vi "Sensors.vi"() -> ()   [LabVIEW 2017]
panel:
  in  "desired temp":dbl
  out "inside":dbl
  out "Gas":dbl
  out "Smoke":dbl
  out "Temp":dbl
  # "Sensors"
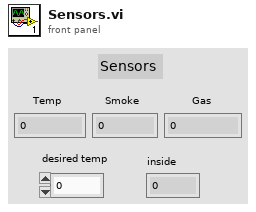
[diagram p1: front panel]
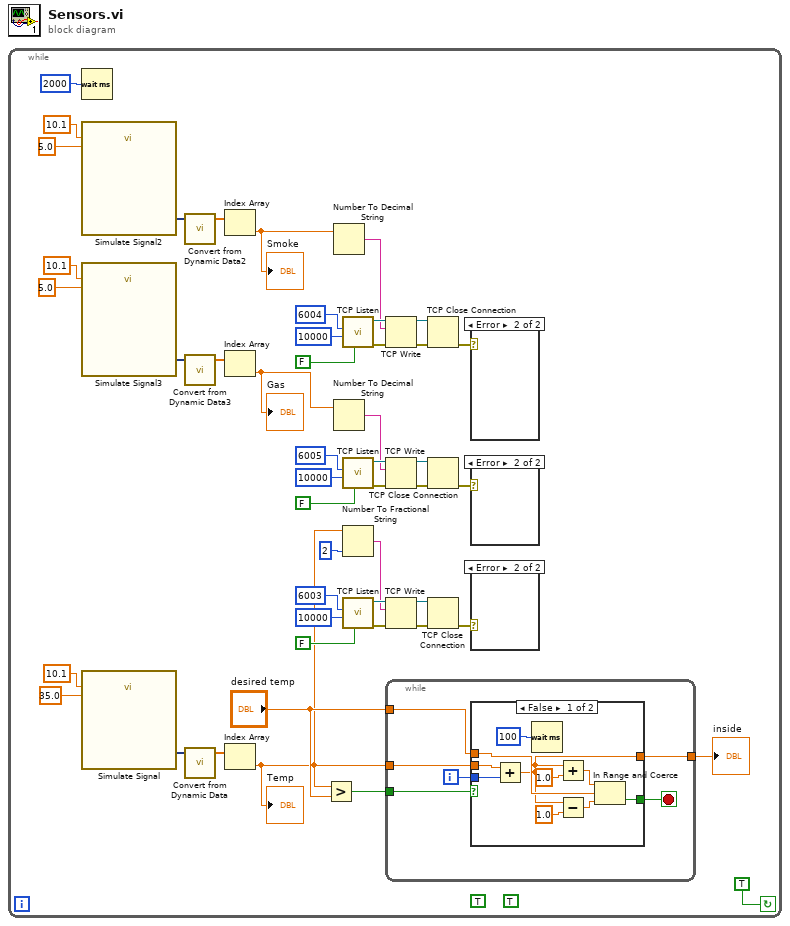
[diagram p0: block diagram]
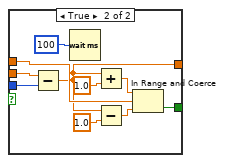
[diagram p5: hidden frame]
diagram:
  n1 = while {
    stop <- TRUE continue-if-true
    (unwired) TRUE
    (unwired) TRUE
    n2 = Wait (ms)(milliseconds to wait=2000) -> ()  [unwired: 1 out]
    n3 = call "Simulate Signal2"("Frequency"=10.1, "Amplitude"=5.0) -> ("Sine"=w32:dynamicdata)  [unwired: 12 in, 1 out]
    n4 = call "Simulate Signal3"("Frequency"=10.1, "Amplitude"=5.0) -> ("Sine"=w19:dynamicdata)  [unwired: 12 in, 1 out]
    n5 = call "Simulate Signal"("Frequency"=10.1, "Amplitude"=35.0) -> ("Sine"=w44:dynamicdata)  [unwired: 12 in, 1 out]
    n6 = call "Convert from Dynamic Data2"("Dynamic Data Type"=w32) -> ("Array"=w31:dbl[])  [unwired: 3 in]
    n7 = call "Convert from Dynamic Data3"("Dynamic Data Type"=w19) -> ("Array"=w18:dbl[])  [unwired: 3 in]
    n8 = call "Convert from Dynamic Data"("Dynamic Data Type"=w44) -> ("Array"=w43:dbl[])  [unwired: 3 in]
    n9 = Index Array(array=w31) -> (element=w22:dbl)  [unwired: 1 in]
    "Smoke" <- w22
    n10 = Index Array(array=w18) -> (element=w9:dbl)  [unwired: 1 in]
    "Gas" <- w9
    n11 = Index Array(array=w43) -> (element=w6:dbl)  [unwired: 1 in]
    "Temp" <- w6
    n12 = Greater?(x=w6, y="desired temp") -> (0:w8:bool)
    n13 = Number To Decimal String(number=w22) -> (decimal integer string=w23:string)  [unwired: 1 in]
    n14 = Number To Decimal String(number=w9) -> (decimal integer string=w10:string)  [unwired: 1 in]
    n15 = call <vilib>:"TCP Listen.vi"("resolve remote address (T)"=FALSE, "timeout ms (wait forever: -1)"=10000, "port"=6004) -> ("error out"=w29:errorcluster, "connection ID"=w27:refnum<k5>)  [unwired: 4 in, 3 out]
    n16 = call <vilib>:"TCP Listen.vi"("resolve remote address (T)"=FALSE, "timeout ms (wait forever: -1)"=10000, "port"=6005) -> ("error out"=w16:errorcluster, "connection ID"=w14:refnum<k5>)  [unwired: 4 in, 3 out]
    n17 = Number To Fractional String(number=w6, precision (6)=i16 2) -> (F-format string=w35:string)  [unwired: 2 in]
    n18 = call <vilib>:"TCP Listen.vi"("resolve remote address (T)"=FALSE, "timeout ms (wait forever: -1)"=10000, "port"=6003) -> ("error out"=w41:errorcluster, "connection ID"=w39:refnum<k5>)  [unwired: 4 in, 3 out]
    n19 = TCP Write(connection ID=w27, data in=w23, error in (no error)=w29) -> (connection ID out=w26:refnum<k5>, error out=w28:errorcluster)  [unwired: 1 in, 1 out]
    n20 = TCP Write(connection ID=w14, data in=w10, error in (no error)=w16) -> (connection ID out=w13:refnum<k5>, error out=w15:errorcluster)  [unwired: 1 in, 1 out]
    n21 = TCP Write(connection ID=w39, data in=w35, error in (no error)=w41) -> (connection ID out=w38:refnum<k5>, error out=w40:errorcluster)  [unwired: 1 in, 1 out]
    n22 = while {
      tunnel: w6 -> [w54]
      tunnel: "desired temp" -> [w53]
      tunnel: w8 -> [w51]
      tunnel: [w49] -> w5
      i -> [w52]
      stop <- w50 stop-if-true
      n23 = case shown="False" w51 {
        tunnel: w54 -> [w56 w66]
        tunnel: w53 -> [w58 w69]
        tunnel: w52 -> [w57 w68]
        tunnel: [w55 w65] -> w49
        tunnel: [w59 w67] -> w50
        frame False {
          n24 = Add(x=w56, y=w57) -> (x+y=w55:dbl)
          n25 = Wait (ms)(milliseconds to wait=u32 100) -> ()  [unwired: 1 out]
          n26 = Add(x=w55, y=1.0) -> (x+y=w63:dbl)
          n27 = Subtract(x=w55, y=1.0) -> (x-y=w61:dbl)
          n28 = In Range and Coerce(upper limit=w63, x=w58, lower limit=w61) -> (In Range?=w59:bool)  [unwired: 1 out]
        }
        frame True {
          n29 = Subtract(x=w66, y=w68) -> (x-y=w65:dbl)
          n30 = Wait (ms)(milliseconds to wait=u32 100) -> ()  [unwired: 1 out]
          n31 = Add(x=w65, y=1.0) -> (x+y=w73:dbl)
          n32 = Subtract(x=w65, y=1.0) -> (x-y=w71:dbl)
          n33 = In Range and Coerce(upper limit=w73, x=w69, lower limit=w71) -> (In Range?=w67:bool)  [unwired: 1 out]
        }
      }
    }
    "inside" <- w5
    n34 = TCP Close Connection(connection ID=w26, error in (no error)=w28) -> (error out=w2:errorcluster)  [unwired: 1 in, 1 out]
    n35 = TCP Close Connection(connection ID=w13, error in (no error)=w15) -> (error out=w1:errorcluster)  [unwired: 1 in, 1 out]
    n36 = TCP Close Connection(connection ID=w38, error in (no error)=w40) -> (error out=w3:errorcluster)  [unwired: 1 in, 1 out]
    n37 = case shown="Error" w2 {
      frame No Error {
      }
      frame Error {
      }
    }
    n38 = case shown="Error" w1 {
      frame No Error {
      }
      frame Error {
      }
    }
    n39 = case shown="Error" w3 {
      frame No Error {
      }
      frame Error {
      }
    }
  }
